vi "VI Tree.vi"   [LabVIEW 2013, in "Stanford Research CG635.lvlib"]
doc: "This is the instrument driver for the <INSTRUMENT NAME>. The VI Tree displays all the user-callable VIs of the instrument driver in an organized table."
uses:
  <instrlib>/Stanford Research CG635/Stanford Research CG635.lvlib
panel:
  # "(c) 2014 National Instruments.  ALL RIGHTS RESERVED."
  # "SEE DIAGRAM\nFOR VI TREE."
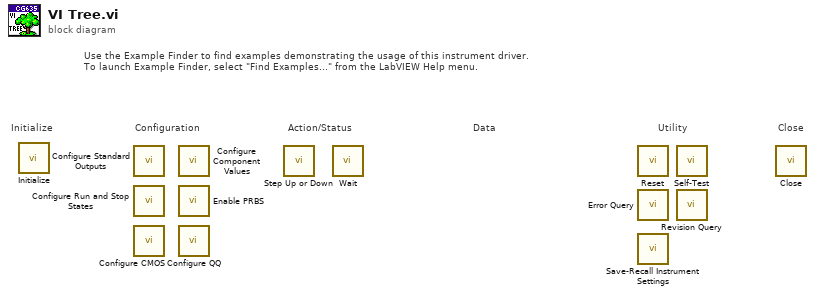
[diagram p0: block diagram]
diagram:
  # "Use the Example Finder to find examples demonstrating the usage of this instrument driver.\nTo launch Example Finder, select \"Find Examples...\" from the LabVIEW Help menu."
  # "Configuration"
  # "Utility"
  # "Data"
  # "Action/Status"
  # "Close"
  # "Initialize"
  n1 = call <instrlib>:"Initialize.vi"() -> ()  [unwired: 10 in, 2 out]
  n2 = call <instrlib>:"Configure Standard Outputs.vi"() -> ()  [unwired: 10 in, 2 out]
  n3 = call <instrlib>:"Configure Run and Stop States.vi"() -> ()  [unwired: 10 in, 2 out]
  n4 = call <instrlib>:"Configure CMOS.vi"() -> ()  [unwired: 10 in, 2 out]
  n5 = call <instrlib>:"Configure Component Values.vi"() -> ()  [unwired: 14 in, 2 out]
  n6 = call <instrlib>:"Enable PRBS.vi"() -> ()  [unwired: 10 in, 2 out]
  n7 = call <instrlib>:"Configure QQ.vi"() -> ()  [unwired: 10 in, 2 out]
  n8 = call <instrlib>:"Step Up or Down.vi"() -> ()  [unwired: 14 in, 2 out]
  n9 = call <instrlib>:"Wait.vi"() -> ()  [unwired: 10 in, 2 out]
  n10 = call <instrlib>:"Reset.vi"() -> ()  [unwired: 10 in, 2 out]
  n11 = call <instrlib>:"Error Query.vi"() -> ()  [unwired: 8 in, 4 out]
  n12 = call <instrlib>:"Save-Recall Instrument Settings.vi"() -> ()  [unwired: 10 in, 2 out]
  n13 = call <instrlib>:"Self-Test.vi"() -> ()  [unwired: 8 in, 4 out]
  n14 = call <instrlib>:"Revision Query.vi"() -> ()  [unwired: 8 in, 4 out]
  n15 = call <instrlib>:"Close.vi"() -> ()  [unwired: 11 in, 1 out]
